vi "串口自动测试.vi"(9 "RS485选择":bool, 11 "RS232选择":bool) -> ()   [LabVIEW 2010]
uses:
  <vilib>/Instr/_visa.llb/VISA Configure Serial Port (Instr).vi
  全局量/试验配置信息.vi
  全局量/自动测试结果.vi
  全局量/全局_配置.vi
panel:
  in  "第2路RS485":string
  in  "第1路RS485":string
  in  "第2路RS232":string
  in  "第1路RS232":string
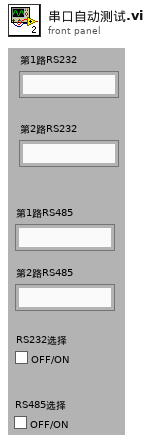
[diagram p1: front panel]
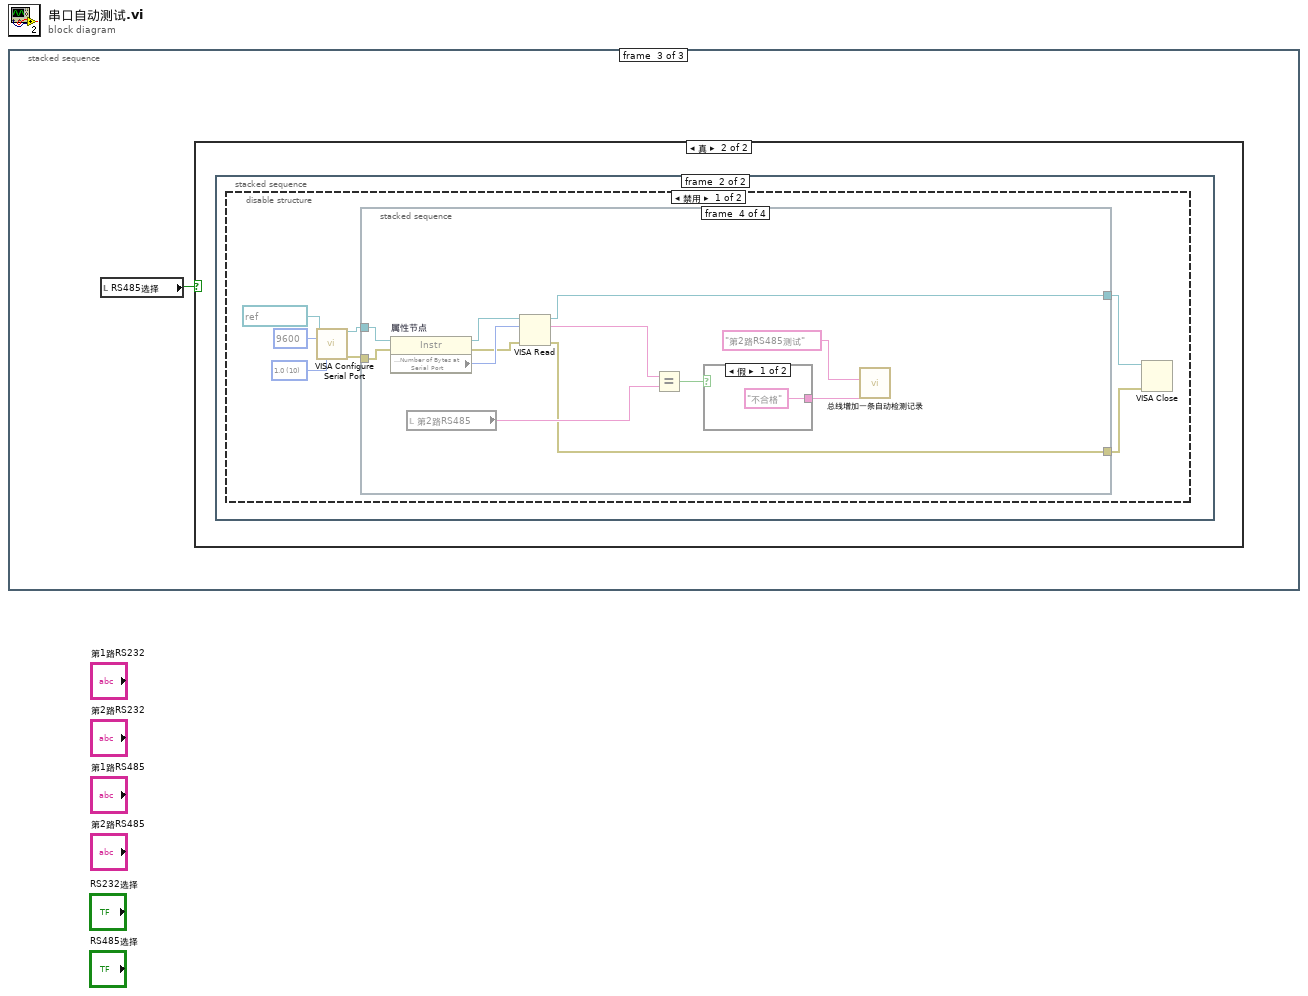
[diagram p0: block diagram]
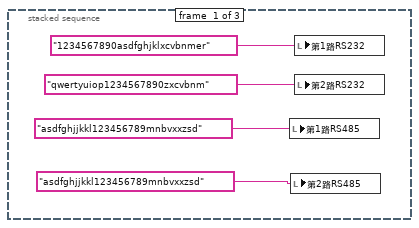
[diagram p2: hidden frame]
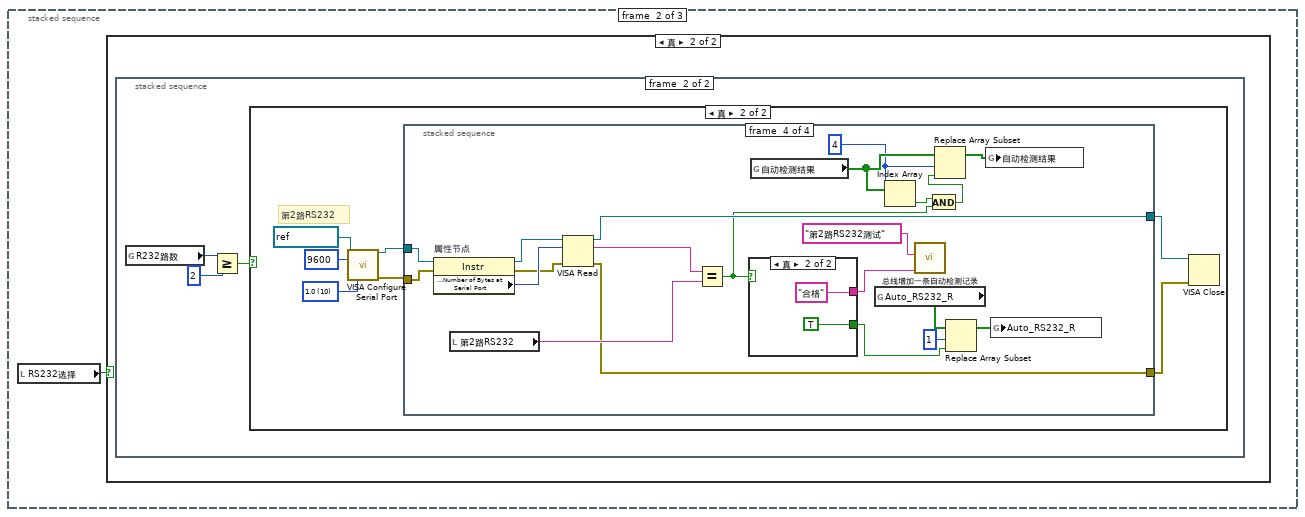
[diagram p3: hidden frame]
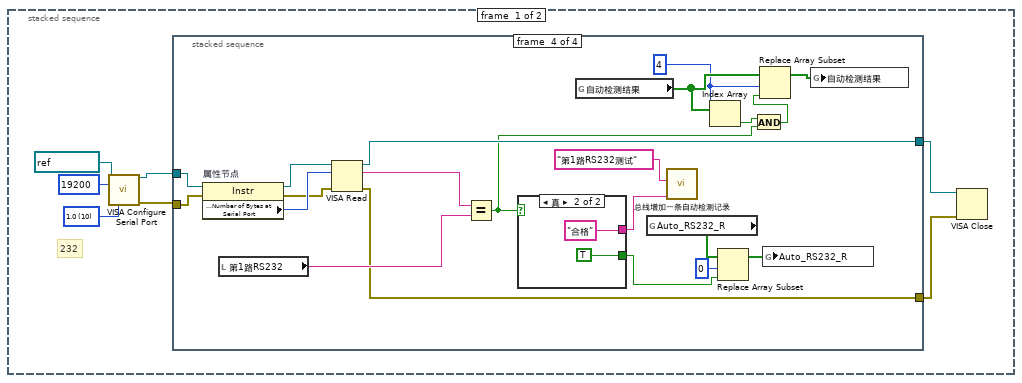
[diagram p5: hidden frame]
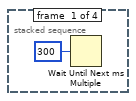
[diagram p6: hidden frame]
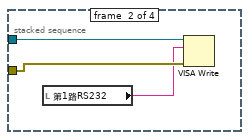
[diagram p7: hidden frame]
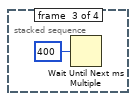
[diagram p8: hidden frame]
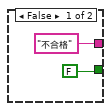
[diagram p9: hidden frame]
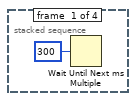
[diagram p11: hidden frame]
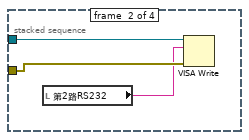
[diagram p12: hidden frame]
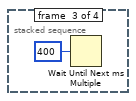
[diagram p13: hidden frame]
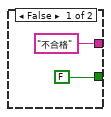
[diagram p14: hidden frame]
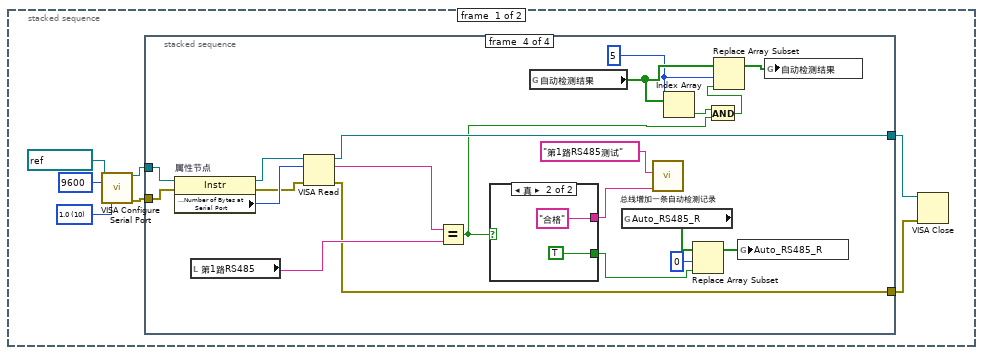
[diagram p16: hidden frame]
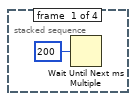
[diagram p17: hidden frame]
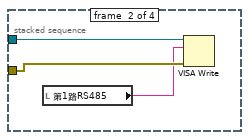
[diagram p18: hidden frame]
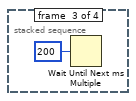
[diagram p19: hidden frame]
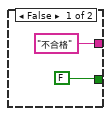
[diagram p20: hidden frame]
diagram:
  n1 = stacked-sequence {
    frame #0 {
      n2 = local write "第1路RS485"("asdfghjjkkl123456789mnbvxxzsd" ("发送字符串_3")) -> ()
      n3 = local write "第2路RS485"("asdfghjjkkl123456789mnbvxxzsd" ("发送字符串_3")) -> ()
      n4 = local write "第1路RS232"("1234567890asdfghjklxcvbnmer" ("发送字符串_1")) -> ()
      n5 = local write "第2路RS232"("qwertyuiop1234567890zxcvbnm" ("发送字符串_2")) -> ()
    }
    frame #1 {
      n6 = local read "RS232选择"() -> (w5:bool)
      n7 = case shown="真" w5 {
        frame False {
        }
        frame True {
          n8 = stacked-sequence {
            frame #0 {
              w8 = u16 10 items=["1.0"=10, "1.5"=15, "2.0"=20] ("stop bits (10: 1 bit)")
              # "232"
              n9 = call-poly "VISA Configure Serial Port"("VISA resource name"=refnum<visa-resource-name> "COM1", "baud rate (9600)"=u32 19200, "stop bits (10: 1 bit)"=w8) -> ("VISA resource name out"=w7:refnum<visa-resource-name>, "error out"=w6:errorcluster)  [unwired: 11 in]
              n10 = stacked-sequence {
                tunnel: w7 -> [_ w16 _ w32]
                tunnel: w6 -> [_ w15 _ w31]
                tunnel: [_ _ _ w34] -> w12
                tunnel: [_ _ _ w33] -> w11
                frame #0 {
                  n11 = Wait Until Next ms Multiple(millisecond multiple=u32 300 ("毫秒倍数")) -> ()  [unwired: 1 out]
                }
                frame #1 {
                  n12 = local read "第1路RS232"() -> (w14:string)
                  n13 = VISA Write(VISA resource name=w16, write buffer=w14, error in (no error)=w15) -> ()  [unwired: 3 out]
                }
                frame #2 {
                  n14 = Wait Until Next ms Multiple(millisecond multiple=u32 400 ("毫秒倍数")) -> ()  [unwired: 1 out]
                }
                frame #3 {
                  w21 = 4 ("索引")
                  n15 = property on="属性节点" class="Instr"(reference=w32, error in=w31) -> (reference out=w38:refnum<visa-resource-name>, error out=w36:errorcluster, "Serial Settings:Number of Bytes at Serial Port"=w37:u32)
                  n16 = local read "第1路RS232"() -> (w35:string)
                  n17 = VISA Read(VISA resource name=w38, byte count=w37, error in (no error)=w36) -> (VISA resource name out=w34:refnum<visa-resource-name>, read buffer=w30:string, error out=w33:errorcluster)  [unwired: 1 out]
                  n18 = Equal?(x=w30, y=w35) -> (x = y?=w19:bool)
                  n19 = case shown="真" w19 {
                    tunnel: ["不合格" "合格"] -> w28
                    tunnel: [FALSE TRUE] -> w24
                    frame False {
                    }
                    frame True {
                    }
                  }
                  n20 = global read "试验配置信息.vi" "自动检测结果"() -> (w22:bool[])
                  n21 = global read "自动测试结果.vi" "Auto_RS232_R"() -> (w27:bool[])
                  n22 = call "总线增加一条自动检测记录.vi"("测试结果"=w28, "测试内容"="第1路RS232测试") -> ()  [unwired: 10 in]
                  n23 = Index Array(array=w22, index=w21) -> (element=w20:bool)
                  n24 = Replace Array Subset(array=w27, new element=w24, index=0 ("索引")) -> (w26:bool[])
                  n25 = And(x=w20, y=w19) -> (x .and. y?=w18:bool)
                  n26 = Replace Array Subset(array=w22, new element=w18, index=w21) -> (w23:bool[])
                  n27 = global write "自动测试结果.vi" "Auto_RS232_R"(w26) -> ()
                  n28 = global write "试验配置信息.vi" "自动检测结果"(w23) -> ()
                }
              }
              n29 = VISA Close(VISA resource name=w12, error in (no error)=w11) -> ()  [unwired: 1 out]
            }
            frame #1 {
              n30 = global read "全局_配置.vi" "R232路数"() -> (w44:u32)
              n31 = Greater Or Equal?(x=w44, y=u32 2) -> (x >= y?=w43:bool)
              n32 = case shown="真" w43 {
                frame False {
                }
                frame True {
                  w48 = u16 10 items=["1.0"=10, "1.5"=15, "2.0"=20] ("stop bits (10: 1 bit)")
                  # "第2路RS232"
                  n33 = call-poly "VISA Configure Serial Port"("VISA resource name"=refnum<visa-resource-name> "COM3", "baud rate (9600)"=u32 9600, "stop bits (10: 1 bit)"=w48) -> ("VISA resource name out"=w51:refnum<visa-resource-name>, "error out"=w52:errorcluster)  [unwired: 11 in]
                  n34 = stacked-sequence {
                    tunnel: w51 -> [_ w56 _ w72]
                    tunnel: w52 -> [_ w55 _ w71]
                    tunnel: [_ _ _ w74] -> w46
                    tunnel: [_ _ _ w73] -> w47
                    frame #0 {
                      n35 = Wait Until Next ms Multiple(millisecond multiple=u32 300 ("毫秒倍数")) -> ()  [unwired: 1 out]
                    }
                    frame #1 {
                      n36 = local read "第2路RS232"() -> (w54:string)
                      n37 = VISA Write(VISA resource name=w56, write buffer=w54, error in (no error)=w55) -> ()  [unwired: 3 out]
                    }
                    frame #2 {
                      n38 = Wait Until Next ms Multiple(millisecond multiple=u32 400 ("毫秒倍数")) -> ()  [unwired: 1 out]
                    }
                    frame #3 {
                      w61 = 4 ("索引")
                      n39 = property on="属性节点" class="Instr"(reference=w72, error in=w71) -> (reference out=w78:refnum<visa-resource-name>, error out=w76:errorcluster, "Serial Settings:Number of Bytes at Serial Port"=w77:u32)
                      n40 = local read "第2路RS232"() -> (w75:string)
                      n41 = VISA Read(VISA resource name=w78, byte count=w77, error in (no error)=w76) -> (VISA resource name out=w74:refnum<visa-resource-name>, read buffer=w68:string, error out=w73:errorcluster)  [unwired: 1 out]
                      n42 = Equal?(x=w68, y=w75) -> (x = y?=w58:bool)
                      n43 = case shown="真" w58 {
                        tunnel: ["不合格" "合格"] -> w69
                        tunnel: [FALSE TRUE] -> w64
                        frame False {
                        }
                        frame True {
                        }
                      }
                      n44 = global read "试验配置信息.vi" "自动检测结果"() -> (w62:bool[])
                      n45 = global read "自动测试结果.vi" "Auto_RS232_R"() -> (w67:bool[])
                      n46 = Index Array(array=w62, index=w61) -> (element=w60:bool)
                      n47 = call "总线增加一条自动检测记录.vi"("测试结果"=w69, "测试内容"="第2路RS232测试") -> ()  [unwired: 10 in]
                      n48 = And(x=w60, y=w58) -> (x .and. y?=w59:bool)
                      n49 = Replace Array Subset(array=w62, new element=w59, index=w61) -> (w63:bool[])
                      n50 = Replace Array Subset(array=w67, new element=w64, index=1 ("索引")) -> (w66:bool[])
                      n51 = global write "试验配置信息.vi" "自动检测结果"(w63) -> ()
                      n52 = global write "自动测试结果.vi" "Auto_RS232_R"(w66) -> ()
                    }
                  }
                  n53 = VISA Close(VISA resource name=w46, error in (no error)=w47) -> ()  [unwired: 1 out]
                }
              }
            }
          }
        }
      }
    }
    frame #2 {
      n54 = local read "RS485选择"() -> (w83:bool)
      n55 = case shown="真" w83 {
        frame False {
        }
        frame True {
          n56 = stacked-sequence {
            frame #0 {
              w88 = u16 10 items=["1.0"=10, "1.5"=15, "2.0"=20] ("stop bits (10: 1 bit)")
              n57 = call-poly "VISA Configure Serial Port"("VISA resource name"=refnum<visa-resource-name> "COM4", "baud rate (9600)"=u32 9600, "stop bits (10: 1 bit)"=w88) -> ("VISA resource name out"=w85:refnum<visa-resource-name>, "error out"=w84:errorcluster)  [unwired: 11 in]
              n58 = stacked-sequence {
                tunnel: w85 -> [_ w94 _ w110]
                tunnel: w84 -> [_ w93 _ w109]
                tunnel: [_ _ _ w112] -> w90
                tunnel: [_ _ _ w111] -> w89
                frame #0 {
                  n59 = Wait Until Next ms Multiple(millisecond multiple=u32 200 ("毫秒倍数")) -> ()  [unwired: 1 out]
                }
                frame #1 {
                  n60 = local read "第1路RS485"() -> (w92:string)
                  n61 = VISA Write(VISA resource name=w94, write buffer=w92, error in (no error)=w93) -> ()  [unwired: 3 out]
                }
                frame #2 {
                  n62 = Wait Until Next ms Multiple(millisecond multiple=u32 200 ("毫秒倍数")) -> ()  [unwired: 1 out]
                }
                frame #3 {
                  w99 = 5 ("索引")
                  n63 = property on="属性节点" class="Instr"(reference=w110, error in=w109) -> (reference out=w116:refnum<visa-resource-name>, error out=w114:errorcluster, "Serial Settings:Number of Bytes at Serial Port"=w115:u32)
                  n64 = local read "第1路RS485"() -> (w113:string)
                  n65 = VISA Read(VISA resource name=w116, byte count=w115, error in (no error)=w114) -> (VISA resource name out=w112:refnum<visa-resource-name>, read buffer=w108:string, error out=w111:errorcluster)  [unwired: 1 out]
                  n66 = Equal?(x=w108, y=w113) -> (x = y?=w96:bool)
                  n67 = case shown="真" w96 {
                    tunnel: ["不合格" "合格"] -> w106
                    tunnel: [FALSE TRUE] -> w102
                    frame False {
                    }
                    frame True {
                    }
                  }
                  n68 = global read "试验配置信息.vi" "自动检测结果"() -> (w100:bool[])
                  n69 = global read "自动测试结果.vi" "Auto_RS485_R"() -> (w105:bool[])
                  n70 = call "总线增加一条自动检测记录.vi"("测试结果"=w106, "测试内容"="第1路RS485测试") -> ()  [unwired: 10 in]
                  n71 = Index Array(array=w100, index=w99) -> (element=w98:bool)
                  n72 = Replace Array Subset(array=w105, new element=w102, index=0 ("索引")) -> (w104:bool[])
                  n73 = And(x=w98, y=w96) -> (x .and. y?=w97:bool)
                  n74 = Replace Array Subset(array=w100, new element=w97, index=w99) -> (w101:bool[])
                  n75 = global write "自动测试结果.vi" "Auto_RS485_R"(w104) -> ()
                  n76 = global write "试验配置信息.vi" "自动检测结果"(w101) -> ()
                }
              }
              n77 = VISA Close(VISA resource name=w90, error in (no error)=w89) -> ()  [unwired: 1 out]
            }
            frame #1 {
              n78 = disable-structure shown="禁用" {
                frame Disabled {
                  w127 = u16 10 items=["1.0"=10, "1.5"=15, "2.0"=20] ("stop bits (10: 1 bit)")
                  n79 = call-poly "VISA Configure Serial Port"("VISA resource name"=refnum<visa-resource-name> "COM5", "baud rate (9600)"=u32 9600, "stop bits (10: 1 bit)"=w127) -> ("VISA resource name out"=w122:refnum<visa-resource-name>, "error out"=w121:errorcluster)  [unwired: 11 in]
                  n80 = stacked-sequence {
                    tunnel: w122 -> [_ w131 _ w137]
                    tunnel: w121 -> [_ w130 _ w136]
                    tunnel: [_ _ _ w139] -> w124
                    tunnel: [_ _ _ w138] -> w123
                    frame #0 {
                      n81 = Wait Until Next ms Multiple(millisecond multiple=u32 200 ("毫秒倍数")) -> ()  [unwired: 1 out]
                    }
                    frame #1 {
                      n82 = local read "第2路RS485"() -> (w129:string)
                      n83 = VISA Write(VISA resource name=w131, write buffer=w129, error in (no error)=w130) -> ()  [unwired: 3 out]
                    }
                    frame #2 {
                      n84 = Wait Until Next ms Multiple(millisecond multiple=u32 200 ("毫秒倍数")) -> ()  [unwired: 1 out]
                    }
                    frame #3 {
                      n85 = property on="属性节点" class="Instr"(reference=w137, error in=w136) -> (reference out=w143:refnum<visa-resource-name>, error out=w141:errorcluster, "Serial Settings:Number of Bytes at Serial Port"=w142:u32)
                      n86 = local read "第2路RS485"() -> (w140:string)
                      n87 = VISA Read(VISA resource name=w143, byte count=w142, error in (no error)=w141) -> (VISA resource name out=w139:refnum<visa-resource-name>, read buffer=w135:string, error out=w138:errorcluster)  [unwired: 1 out]
                      n88 = Equal?(x=w135, y=w140) -> (x = y?=w144:bool)
                      n89 = case shown="假" w144 {
                        tunnel: ["不合格" "合格"] -> w133
                        frame False {
                        }
                        frame True {
                        }
                      }
                      n90 = call "总线增加一条自动检测记录.vi"("测试结果"=w133, "测试内容"="第2路RS485测试") -> ()  [unwired: 10 in]
                    }
                  }
                  n91 = VISA Close(VISA resource name=w124, error in (no error)=w123) -> ()  [unwired: 1 out]
                }
                frame Enabled {
                }
              }
            }
          }
        }
      }
    }
  }
